vi "test cluster channels for configure cases.vi"() -> ()   [LabVIEW 2020]
uses:
  BaseDriver/DriverMsg.ctl
panel:
  in  "Msg in":T1={"Command"="setPosition.Axis 1", "Args"=["23.5"]}
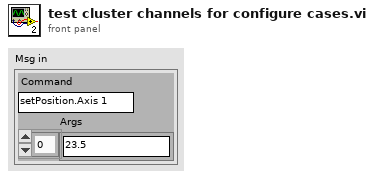
[diagram p1: front panel]
types:
  T1 = typedef "DriverMsg.ctl" = cluster{"Command":string, "Args":string[]}
  T2 = typedef "parsed device cmd.ctl" = cluster{"Command":string, "Args":string[], "Seperator in":string}
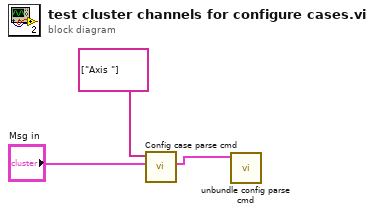
[diagram p0: block diagram]
diagram:
  n1 = call "Config case parse cmd.vi"("Msg in"="Msg in", "Seperator"=string[] ["Axis "]) -> ("Parsed CMD"=w1:T2)  [unwired: 8 in, 1 out]
  n2 = call "unbundle config parse cmd.vi"("Parsed CMD"=w1) -> ()  [unwired: 7 in, 4 out]
